vi "Assign Point Ramping (beta).vi"(5 "Ramp Time [sec]":dbl=3.0, 6 "L1 to L4 PID Cluster":T1={"L1 PID Gains"={"Kp"=0.005, "Kd"=0.5, "Ki"=0.0005}, "L2 PID Gains"={"Kp"=0.01, "Kd"=1.0, "Ki"=0.0005}, "L3 PID Gains"={"Kp"=0.05, "Kd"=1.0, "Ki"=0.0005}, "L4 PID Gains"={"Kp"=0.1, "Kd"=0.1, "Ki"=0.0005}}, 7 "Offset Home2RCM":dbl[](array[numeric])=[0.0, 0.0, 0.0, 0.0], 8 "Destination Posit Array [mm]":dbl[](array[numeric])=[0.0, 0.0, -3.0, 0.0], 9 "Previous Posit Array":dbl[](array[numeric])=[0.0, 0.0, 0.0, 0.0], 10 "error in":errorcluster, 11 "FPGA VI Reference In":refnum<k20>) -> (1 "Last L1 to L4 Posit":dbl[](array[numeric]), 2 "error out":errorcluster, 3 "FPGA VI Reference Out":refnum<k20>)   [LabVIEW 2016]
uses:
  <vilib>/Analysis/1siggen.llb/Ramp Pattern by Samples.vi
  Subsystems/Global Variables.vi
  <vilib>/Analysis/NI_AALBase.lvlib
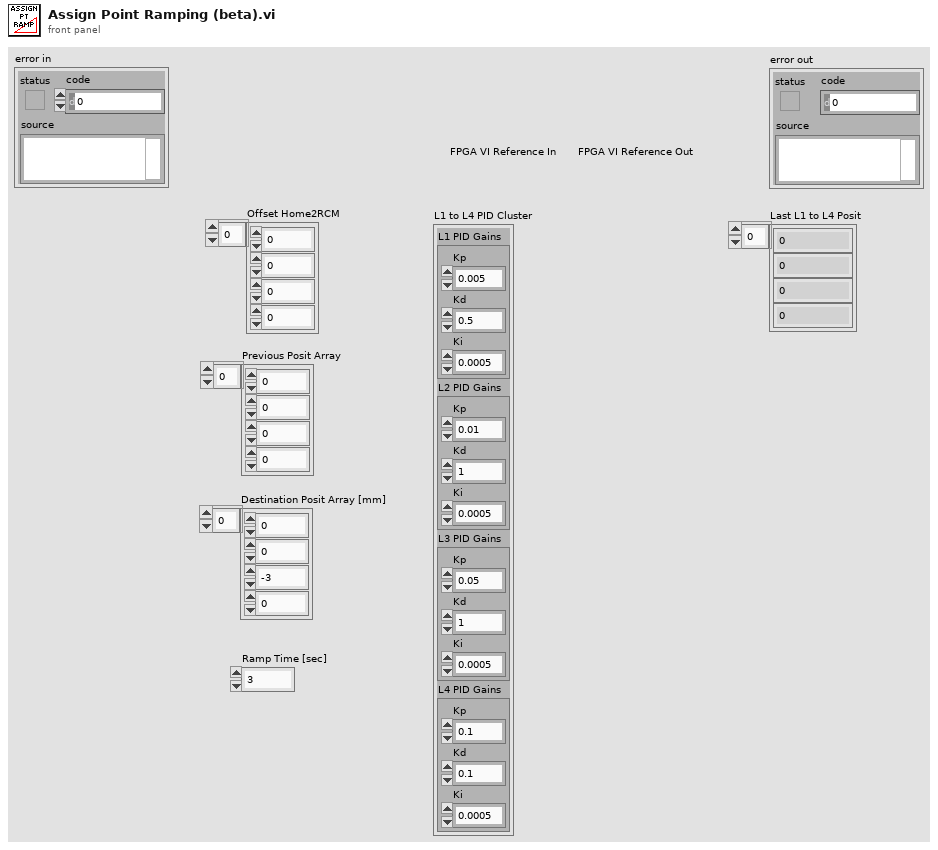
[diagram p1: front panel]
types:
  T1 = cluster{"L1 PID Gains":cluster{"Kp":dbl, "Kd":dbl, "Ki":dbl}, "L2 PID Gains":cluster{"Kp":dbl, "Kd":dbl, "Ki":dbl}, "L3 PID Gains":cluster{"Kp":dbl, "Kd":dbl, "Ki":dbl}, "L4 PID Gains":cluster{"Kp":dbl, "Kd":dbl, "Ki":dbl}}
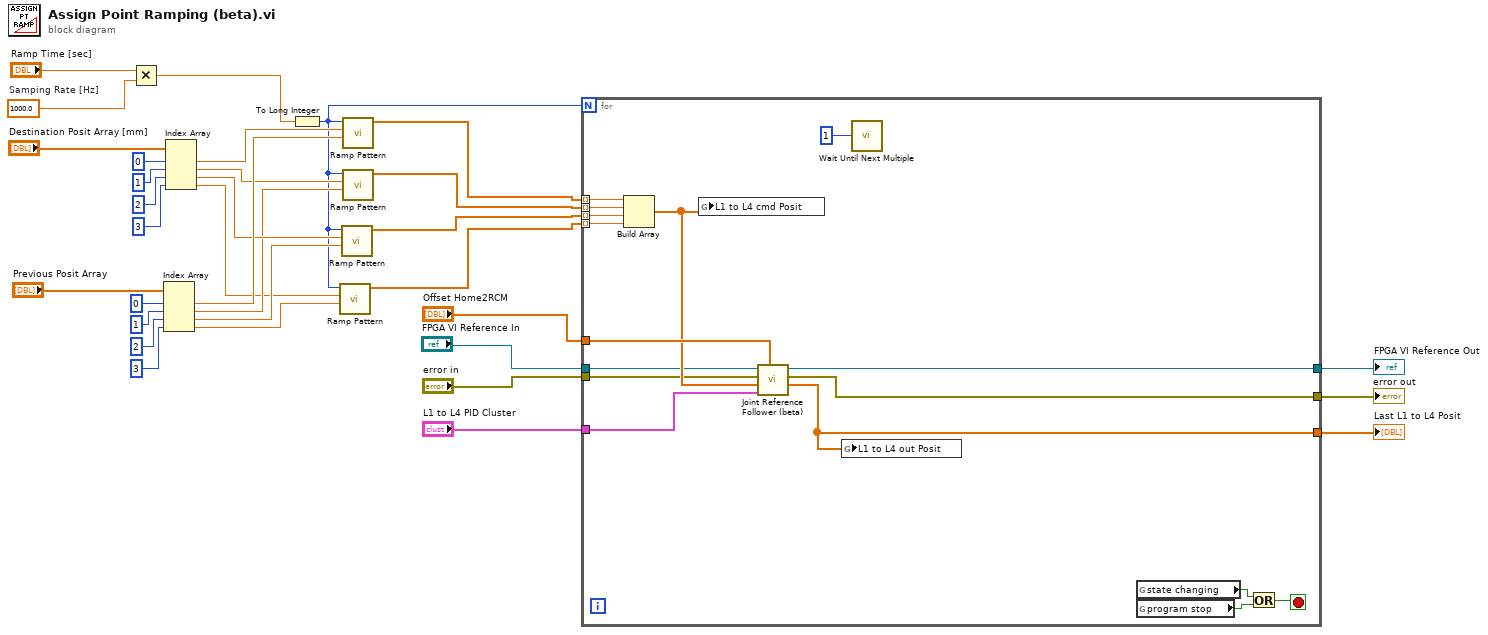
[diagram p0: block diagram]
diagram:
  w22 = 1000.0  # Samping Rate [Hz]
  n1 = Multiply(x="Ramp Time [sec]", y=w22) -> (x*y=w13:dbl)
  n2 = Index Array(array="Previous Posit Array", index #1=0 ("index"), index #2=1 ("index"), index #3=2 ("index"), index #4=3 ("index")) -> (element #1=w21:dbl, element #2=w17:dbl, element #3=w16:dbl, element #4=w15:dbl)
  n3 = Index Array(array="Destination Posit Array [mm]", index #1=0 ("index"), index #2=1 ("index"), index #3=2 ("index"), index #4=3 ("index")) -> (element #1=w20:dbl, element #2=w19:dbl, element #3=w18:dbl, element #4=w14:dbl)
  n4 = To Long Integer(number=w13) -> (32bit integer=w12:i32)
  n5 = call-poly <vilib>:"Ramp Pattern.vi"("start"=w15, "end"=w14, "samples"=w12) -> ("Ramp Pattern"=w8:dbl[])  [unwired: 7 in, 1 out]
  n6 = call-poly <vilib>:"Ramp Pattern.vi"("start"=w16, "end"=w18, "samples"=w12) -> ("Ramp Pattern"=w9:dbl[])  [unwired: 7 in, 1 out]
  n7 = call-poly <vilib>:"Ramp Pattern.vi"("start"=w21, "end"=w20, "samples"=w12) -> ("Ramp Pattern"=w11:dbl[])  [unwired: 7 in, 1 out]
  n8 = call-poly <vilib>:"Ramp Pattern.vi"("start"=w17, "end"=w19, "samples"=w12) -> ("Ramp Pattern"=w10:dbl[])  [unwired: 7 in, 1 out]
  n9 = for {
    N: w12 -> [_]
    tunnel: w11 -> [w49] mode=indexing
    tunnel: w10 -> [w48] mode=indexing
    tunnel: w9 -> [w47] mode=indexing
    tunnel: w8 -> [w46] mode=indexing
    tunnel: [w45] -> w1
    tunnel: [w44] -> w4
    tunnel: "Offset Home2RCM" -> [w43]
    tunnel: "L1 to L4 PID Cluster" -> [w42]
    tunnel: [w40] -> w6
    tunnel: "FPGA VI Reference In" -> [w38]
    tunnel: "error in" -> [w37]
    stop <- w34 stop-if-true
    n10 = Build Array(w49, w48, w47, w46) -> (w41:dbl[])
    n11 = global write "Global Variables.vi" "L1 to L4 cmd Posit"(w41) -> ()
    n12 = call "Joint Reference Follower (beta).vi"("Offset Home2RCM [deg/mm]"=w43, "PID Ctrl Cluster"=w42, "Ref Array [deg/mm]"=w41, "error in"=w37, "FPGA VI Reference In"=w38) -> ("Output Posit Array [deg/mm]"=w40:dbl[], "error out"=w44:errorcluster, "FPGA VI Reference Out"=w45:refnum<k20>)  [unwired: 4 in]
    n13 = global write "Global Variables.vi" "L1 to L4 out Posit"(w40) -> ()
    n14 = call "Wait Until Next Multiple"("Count(mSec)"=u32 1) -> ()  [unwired: 1 out]
    n15 = global read "Global Variables.vi" "state changing"() -> (w36:bool)
    n16 = global read "Global Variables.vi" "program stop"() -> (w35:bool)
    n17 = Or(x=w36, y=w35) -> (x .or. y?=w34:bool)
  }
  "error out" <- w4
  "Last L1 to L4 Posit" <- w6
  "FPGA VI Reference Out" <- w1
